vi "IT6724C_Config.vi"(7 "等待时间(毫秒)":u32=100, 8 "error in":errorcluster caption="错误输入（无错误）", 9 "数值":dbl=15.0, 10 "电压电流":enum16{"VOLTage", "CURR"}(ring), 11 "MyIndex":u8) -> (0 "error out":errorcluster, 3 "返回值":string)   [LabVIEW 2015, in "IT6724.lvlib"]
uses:
  IT6724.lvlib
  <vilib>/Instr/_visa.llb/VISA Configure Serial Port (Instr).vi
panel:
  out "VISA":refnum<visa-resource-name>
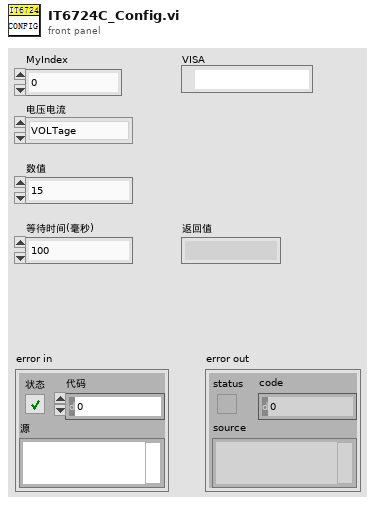
[diagram p1: front panel]
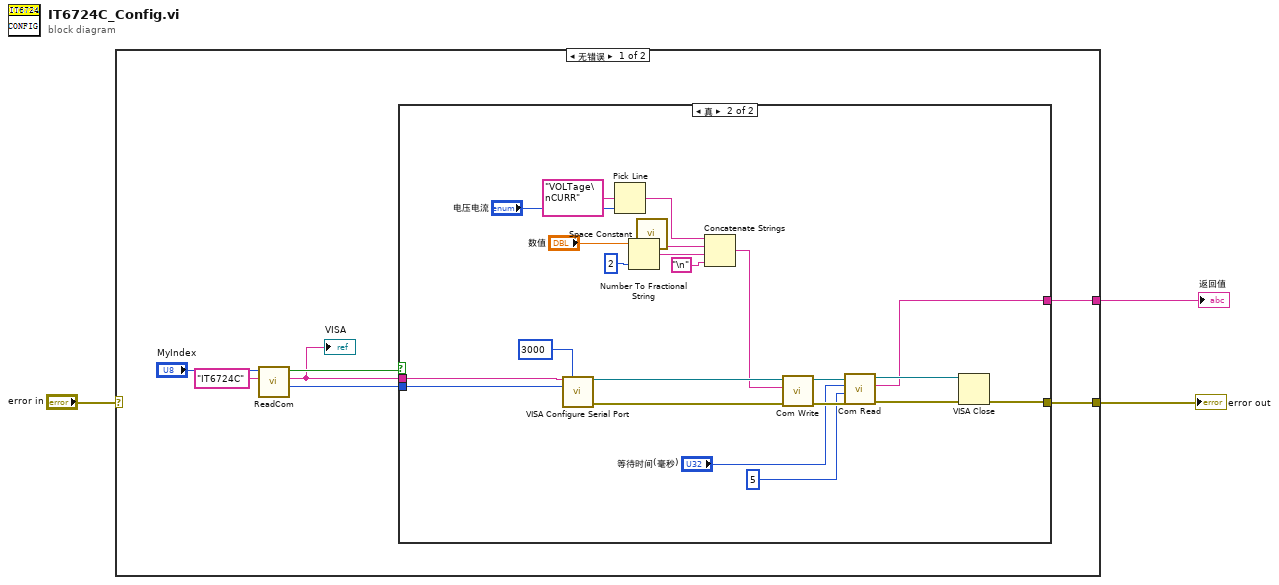
[diagram p0: block diagram]
diagram:
  n1 = case shown="无错误" "error in" {
    selector: "error in" -> [_ w33]
    tunnel: [w10 w33] -> w3
    tunnel: [w4 _] -> w1
    frame No Error {
      n2 = call "ReadCom.vi"("仪器名称"="IT6724C", "MyIndex"="MyIndex") -> ("Baudrate"=w5:i32, "COM"=w6:string, "OK?"=w7:bool)  [unwired: 7 in]
      "VISA" <- w6
      n3 = case shown="真" w7 {
        tunnel: [_ w32] -> w10
        tunnel: w6 -> [_ w31]
        tunnel: w5 -> [_ w30]
        tunnel: [_ w22] -> w4
        frame False {
        }
        frame True {
          n4 = call-poly "VISA Configure Serial Port"("VISA resource name"=w31, "timeout (10sec)"=u32 3000, "baud rate (9600)"=w30) -> ("VISA resource name out"=w28:refnum<visa-resource-name>, "error out"=w27:errorcluster)  [unwired: 11 in]
          n5 = Pick Line(multi-line string="VOLTage\nCURR", line index="电压电流") -> (output string=w21:string)  [unwired: 1 in]
          n6 = Number To Fractional String(number="数值", precision (6)=i16 2 ("精度(6)")) -> (F-format string=w16:string)  [unwired: 2 in]
          n7 = call <vilib>:"Space Constant.vi"() -> ("String"=w15:string)
          n8 = Concatenate Strings(w21, w15, w16, "\n") -> (w13:string)
          n9 = call "Com Write.vi"("错误输入（无错误）"=w27, "Wbuff"=w13, "VISA In"=w28) -> ("错误输出"=w25:errorcluster, "VISA Out"=w26:refnum<visa-resource-name>)  [unwired: 7 in]
          n10 = call "Com Read.vi"("错误输入（无错误）"=w25, "num"=u32 5, "超时"="等待时间(毫秒)", "VISA In"=w26) -> ("错误输出"=w24:errorcluster, "buff"=w22:string, "VISA Out"=w23:refnum<visa-resource-name>)  [unwired: 5 in]
          n11 = VISA Close(VISA resource name=w23, error in (no error)=w24) -> (error out=w32:errorcluster)
        }
      }
    }
    frame Error {
    }
  }
  "error out" <- w3
  "返回值" <- w1
